vi "DiagramToJson.vi"(5 "Owner Bounds":T1, 6 "Origin Path":path, 7 "Image Path":path, 8 "error in (no error)":errorcluster, 9 "Current Path":path, 10 "ID":string, 11 "GObj in":refnum<vi>) -> (0 "error out":errorcluster, 1 "JSON (out)":string, 3 "GObj out":refnum<vi>)   [LabVIEW 2017]
doc: "Creates JSON for a diagram objectaJSON generator for Finale.\nInput: \nDiagram: Diagram in\nBlock diagram in case of top level, else normal diagram.\n\nCurrent Path: String\nControls the current path in the tree\n\nOrigin Path:\nContains the root directory, sub-VIs\n\nOutput:\nJSON String: String\nIndicates the json string for Diagram"
uses:
  <vilib>/Utility/miscctls.llb/LVRectTypeDef.ctl
  GObjectConverters/SubVIConverter/SubVIConverter.lvclass
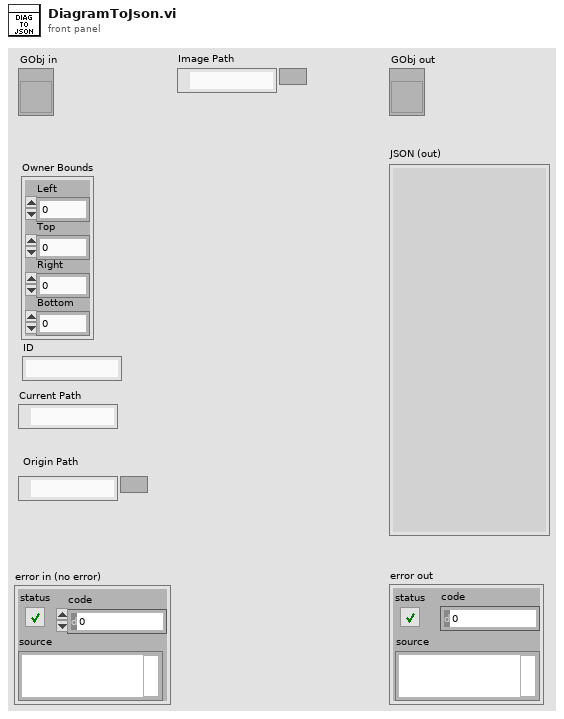
[diagram p1: front panel]
types:
  T1 = typedef "LVRectTypeDef.ctl" = cluster{"Left":i16, "Top":i16, "Right":i16, "Bottom":i16}
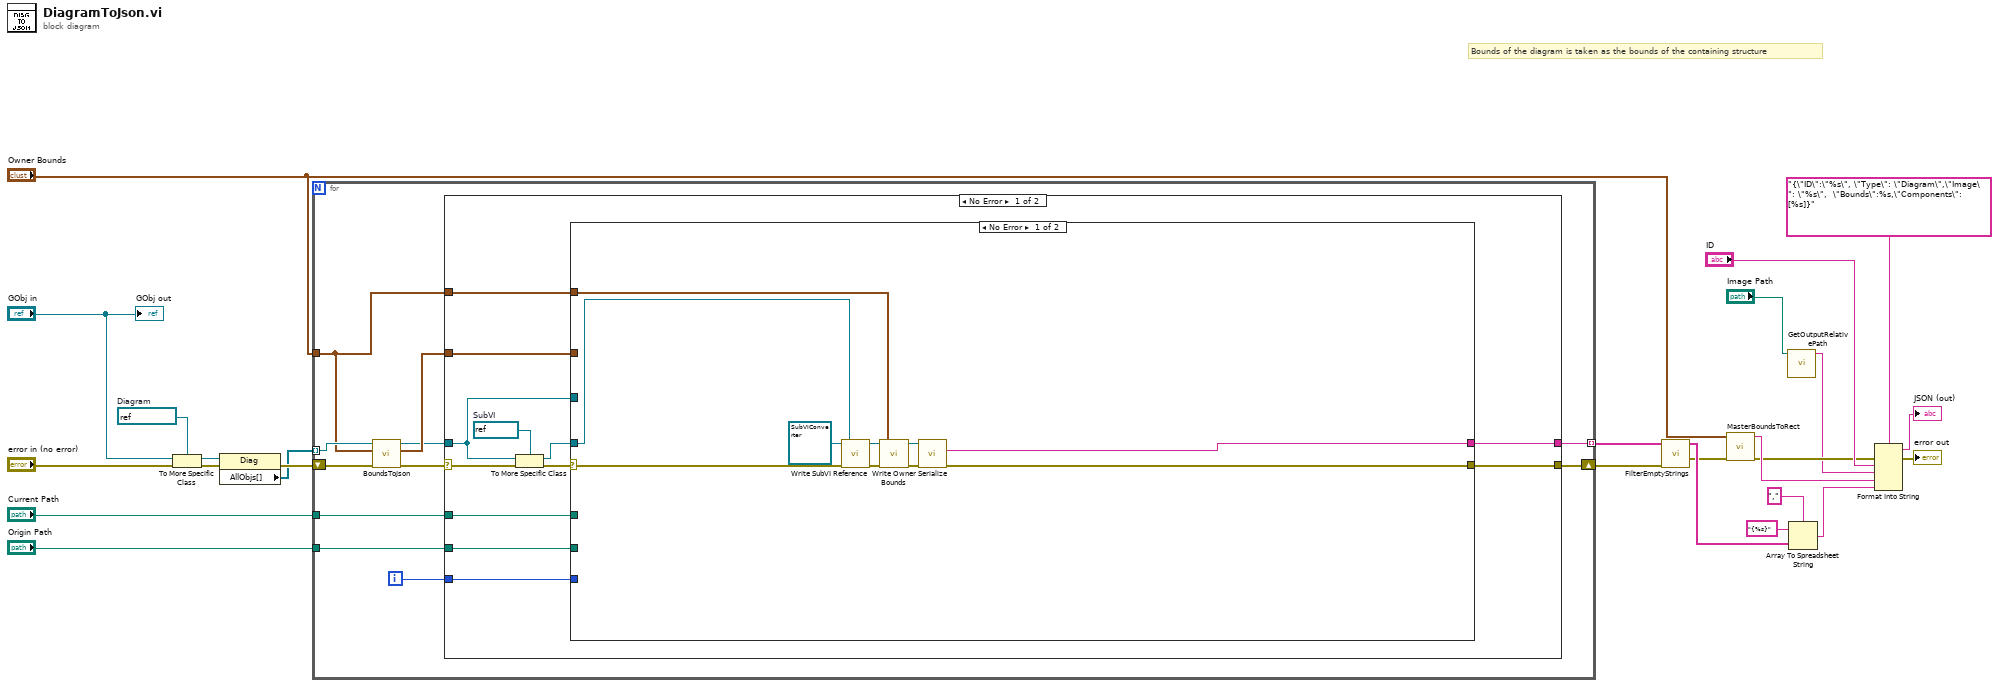
[diagram p0: block diagram]
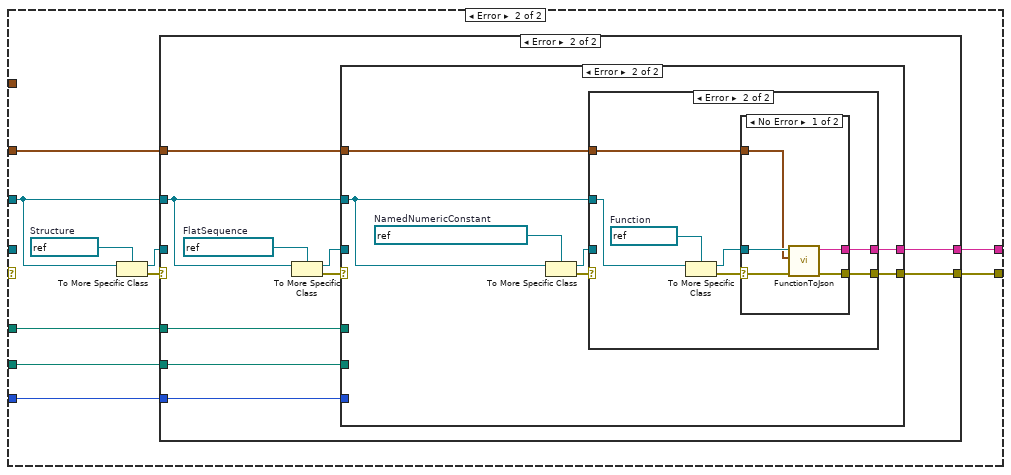
[diagram p2: hidden frame]
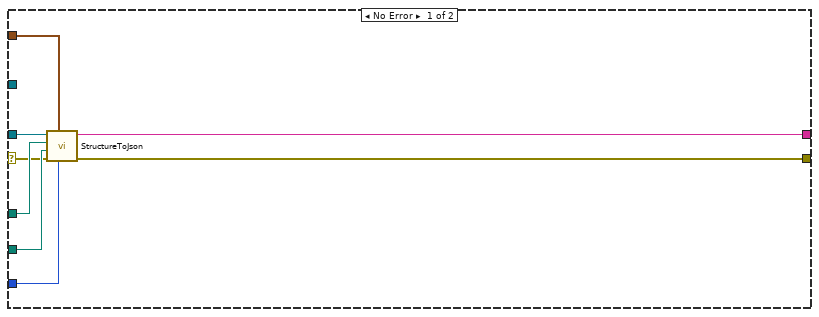
[diagram p3: hidden frame]
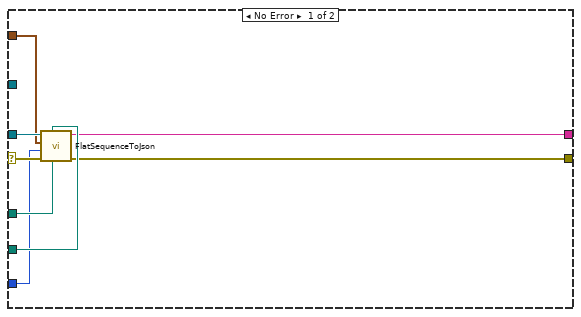
[diagram p4: hidden frame]
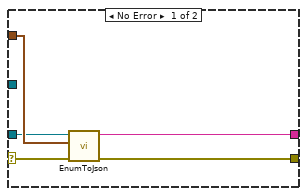
[diagram p5: hidden frame]
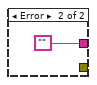
[diagram p6: hidden frame]
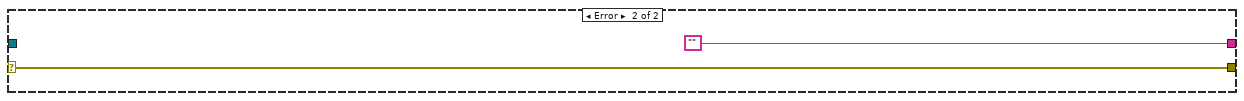
[diagram p7: hidden frame]
diagram:
  w18 = refnum<vi> refnum  # Diagram
  # "Bounds of the diagram is taken as the bounds of the containing structure"
  n1 = To More Specific Class(target class=w18, reference="GObj in", error in="error in (no error)") -> (specific class reference=w19:refnum<vi>, error out=w16:errorcluster)
  n2 = property class="Diag"(reference=w19, error in=w16) -> (error out=w21:errorcluster, "AllObjs[]"=w3:refnum<vi>[])  [unwired: 1 out]
  n3 = for {
    tunnel: w3 -> [w35] mode=indexing
    tunnel: [w33] -> w25 mode=indexing
    tunnel: "Owner Bounds" -> [w26]
    shift-right: [w34] -> w20
    shift-left: w21 -> [w36]
    tunnel: "Current Path" -> [w31]
    tunnel: "Origin Path" -> [w30]
    i -> [w29]
    n4 = call "BoundsToJson.vi"("error in (no error)"=w36, "Owner Bounds"=w26, "GObj in"=w35) -> ("error out"=w27:errorcluster, "Relative Bounds"=w32:cluster{"x":i32, "y":i32, "w":i32, "h":i32}, "GObj out"=w28:refnum<vi>)  [unwired: 5 in, 1 out]
    n5 = case shown="No Error" w27 {
      selector: w27 -> [w38 w121]
      tunnel: [w46 w121] -> w34
      tunnel: [w45 ""] -> w33
      tunnel: w32 -> [w44 _]
      tunnel: w31 -> [w43 _]
      tunnel: w30 -> [w42 _]
      tunnel: w29 -> [w41 _]
      tunnel: w28 -> [w40 _]
      tunnel: w26 -> [w37 _]
      frame No Error {
        w47 = refnum<vi> refnum  # SubVI
        n6 = To More Specific Class(target class=w47, reference=w40, error in=w38) -> (specific class reference=w39:refnum<vi>, error out=w48:errorcluster)
        n7 = case shown="No Error" w48 {
          selector: w48 -> [w53 _]
          tunnel: w44 -> [_ w64]
          tunnel: [w50 w62] -> w46
          tunnel: [w51 w59] -> w45
          tunnel: w43 -> [_ w67]
          tunnel: w42 -> [_ w66]
          tunnel: w41 -> [_ w65]
          tunnel: w40 -> [_ w60]
          tunnel: w39 -> [w57 _]
          tunnel: w37 -> [w55 _]
          frame No Error {
            n8 = call-dynamic "Write SubVI Reference.vi"("error in (no error)"=w53, "SubVI Reference"=w57, "SubVIConverter in"=refnum<class "SubVIConverter.lvclass"> refnum ("SubVIConverter.lvclass")) -> ("error out"=w54:errorcluster, "SubVIConverter out"=w56:refnum<class "SubVIConverter.lvclass">)  [unwired: 7 in]
            n9 = call-dynamic "Write Owner Bounds.vi"("error in (no error)"=w54, "Rect"=w55, "VIObjectConverter in"=w56) -> ("error out"=w49:errorcluster, "VIObjectConverter out"=w52:refnum<class "SubVIConverter.lvclass">)  [unwired: 7 in]
            n10 = call-dynamic "Serialize.vi"("error in (no error)"=w49, "SubVIConverter in"=w52) -> ("error out"=w50:errorcluster, "JSON"=w51:string)  [unwired: 7 in, 1 out]
          }
          frame Error {
            w63 = refnum<vi> refnum  # Structure
            n11 = To More Specific Class(target class=w63, reference=w60) -> (specific class reference=w61:refnum<vi>, error out=w68:errorcluster)  [unwired: 1 in]
            n12 = case shown="Error" w68 {
              selector: w68 -> [w71 _]
              tunnel: w64 -> [w76 w79]
              tunnel: w67 -> [w75 w81]
              tunnel: w66 -> [w74 w82]
              tunnel: w65 -> [w73 w80]
              tunnel: [w72 w83] -> w62
              tunnel: w61 -> [w70 _]
              tunnel: w60 -> [_ w78]
              tunnel: [w69 w77] -> w59
              frame No Error {
                n13 = call "StructureToJson.vi"("Component Idx"=w73, "Relative Bounds"=w76, "error in (no error)"=w71, "Origin Path"=w74, "Current Path"=w75, "GObj (in)"=w70) -> ("error out"=w72:errorcluster, "JSON"=w69:string)  [unwired: 4 in]
              }
              frame Error {
                w86 = refnum<vi> refnum  # FlatSequence
                n14 = To More Specific Class(target class=w86, reference=w78) -> (specific class reference=w84:refnum<vi>, error out=w85:errorcluster)  [unwired: 1 in]
                n15 = case shown="Error" w85 {
                  selector: w85 -> [w93 _]
                  tunnel: w84 -> [w94 _]
                  tunnel: [w87 w101] -> w77
                  tunnel: [w88 w100] -> w83
                  tunnel: w82 -> [w92 _]
                  tunnel: w81 -> [w91 _]
                  tunnel: w80 -> [w90 _]
                  tunnel: w79 -> [w89 w98]
                  tunnel: w78 -> [_ w95]
                  frame No Error {
                    n16 = call "FlatSequenceToJson.vi"("Current Path"=w91, "Origin Path"=w92, "error in"=w93, "Component Idx"=w90, "Relative Bounds"=w89, "FlatSequence in"=w94) -> ("error out"=w88:errorcluster, "JSON"=w87:string)  [unwired: 4 in]
                  }
                  frame Error {
                    w97 = refnum<vi> refnum  # NamedNumericConstant
                    n17 = To More Specific Class(target class=w97, reference=w95) -> (specific class reference=w99:refnum<vi>, error out=w96:errorcluster)  [unwired: 1 in]
                    n18 = case shown="Error" w96 {
                      selector: w96 -> [w106 _]
                      tunnel: [w103 w109] -> w100
                      tunnel: [w102 w107] -> w101
                      tunnel: w99 -> [w104 _]
                      tunnel: w98 -> [w105 w108]
                      tunnel: w95 -> [_ w113]
                      frame No Error {
                        n19 = call "EnumToJson.vi"("error in"=w106, "Relative Bounds"=w105, "GObj in"=w104) -> ("error out"=w103:errorcluster, "JSON"=w102:string)  [unwired: 7 in]
                      }
                      frame Error {
                        w112 = refnum<vi> refnum  # Function
                        n20 = To More Specific Class(target class=w112, reference=w113) -> (specific class reference=w110:refnum<vi>, error out=w111:errorcluster)  [unwired: 1 in]
                        n21 = case shown="No Error" w111 {
                          selector: w111 -> [w116 _]
                          tunnel: w110 -> [w118 _]
                          tunnel: [w115 _] -> w109
                          tunnel: w108 -> [w117 _]
                          tunnel: [w114 ""] -> w107
                          frame No Error {
                            n22 = call "FunctionToJson.vi"("error in (no error)"=w116, "Relative Bounds"=w117, "Function Ref In"=w118) -> ("error out"=w115:errorcluster, "JSON"=w114:string)  [unwired: 7 in]
                          }
                          frame Error {
                          }
                        }
                      }
                    }
                  }
                }
              }
            }
          }
        }
      }
      frame Error {
      }
    }
  }
  n23 = call "FilterEmptyStrings.vi"("error in"=w20, "Array in"=w25) -> ("error out"=w6:errorcluster, "Array out"=w24:string[])  [unwired: 8 in]
  n24 = call "MasterBoundsToRect.vi"("error in"=w6, "Owner Bounds"="Owner Bounds") -> ("error out"=w7:errorcluster, "JSON"=w8:string)  [unwired: 8 in]
  n25 = call "GetOutputRelativePath.vi"("Path"="Image Path") -> ("Output relative path"=w1:string)  [unwired: 9 in, 1 out]
  n26 = Array To Spreadsheet String(delimiter (Tab)=",", array=w24, 3:"{%s}" ("format string")) -> (spreadsheet string=w13:string)
  n27 = Format Into String(format string="{\"ID\":\"%s\", \"Type\": \"Diagram\",\"Image\": \"%s\",  \"Bounds\":%s,\"Components\": [%s]}", error in=w7, "ID", w1, w8, w13) -> (resulting string=→"JSON (out)":string, error out=→"error out":errorcluster)  [unwired: 1 in]
  "GObj out" <- "GObj in"
